vi "brace_tare_file_stream.vi"(11 "Sensor Output (mm)":dbl[][][](array[numeric])) -> (3 "Tared Sensor Output - Position (mm)":dbl[][][](array[numeric]))   [LabVIEW 2018]
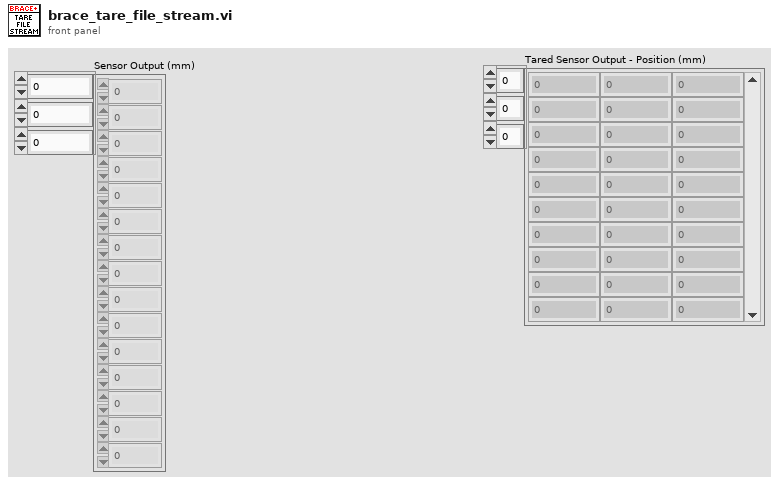
[diagram p1: front panel]
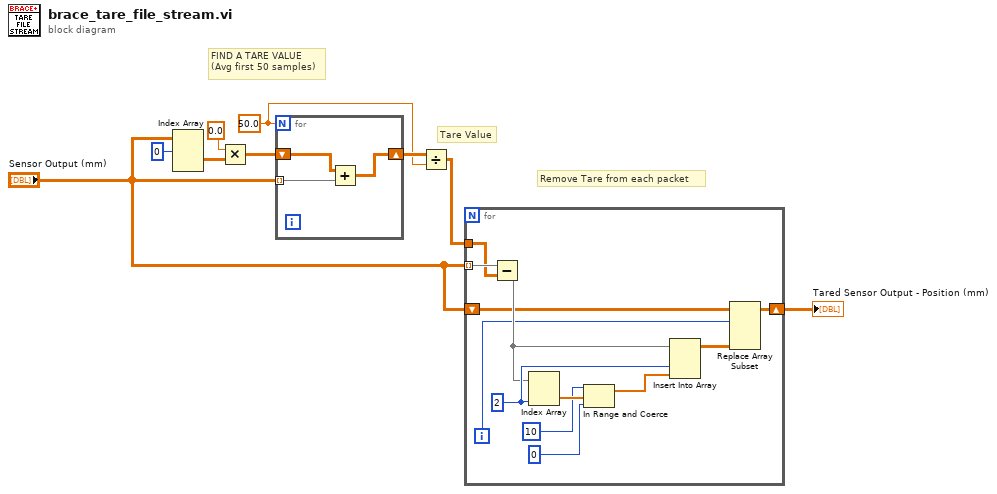
[diagram p0: block diagram]
diagram:
  w4 = 50.0
  # "Remove Tare from each packet"
  # "Tare Value"
  # "FIND A TARE VALUE\n(Avg first 50 samples)"
  n1 = Index Array(array="Sensor Output (mm)", index (dim 0)=0 ("index (page)")) -> (element=w7:dbl[][])  [unwired: 2 in]
  n2 = Multiply(x=0.0, y=w7) -> (x*y=w8:dbl[][])
  n3 = for {
    N: w4 -> [_]
    tunnel: "Sensor Output (mm)" -> [w11] mode=indexing
    shift-right: [w10] -> w5
    shift-left: w8 -> [w12]
    n4 = Add(x=w12, y=w11) -> (x+y=w10:dbl[][])
  }
  n5 = Divide(x=w5, y=w4) -> (x/y=w3:dbl[][])
  n6 = for {
    tunnel: "Sensor Output (mm)" -> [w23] mode=indexing
    tunnel: w3 -> [w22]
    shift-right: [w17] -> w1
    shift-left: "Sensor Output (mm)" -> [w19]
    i -> [w18]
    w24 = 2 ("disabled index (col)")
    n7 = Subtract(x=w23, y=w22) -> (x-y=w20:dbl[][])
    n8 = Index Array(array=w20, index (col)=w24) -> (element=w21:dbl[])  [unwired: 1 in]
    n9 = In Range and Coerce(upper limit=10, x=w21, lower limit=0) -> (coerced(x)=w14:dbl[])  [unwired: 1 out]
    n10 = Insert Into Array(array=w20, index (col)=w24, new element=w14) -> (w13:dbl[][])  [unwired: 1 in]
    n11 = Replace Array Subset(array=w19, new element=w13, index (dim 0)=w18) -> (w17:dbl[][][])  [unwired: 2 in]
  }
  "Tared Sensor Output - Position (mm)" <- w1
